vi "Get All Process Names.vi"(11 "?":T16 {"Main Config"."PR Module Configs"."Settings"."PID 2 Parameters"."output range"."output low" format="%.2f"; "Main Config"."PR Module Configs"."Settings"."PID 2 Parameters"."output range"."output high" min=0.0 max=100.0 format="%.2f"; "Main Config"."PR Module Configs"."Settings"."PID 2 Parameters"."PID gains"."derivative time (Td, min)" format="%.3f"; "Main Config"."PR Module Configs"."Settings"."PID 2 Parameters"."PID gains"."integral time (Ti, min)" format="%.3f"; "Main Config"."PR Module Configs"."Settings"."PID 2 Parameters"."PID gains"."proportional gain (Kc)" format="%.3f"; "Main Config"."Steps"."Control" items=["Pump %", "Setpoint"]; "Main Config"."TCU Module Configs"."Settings"."Huber Unistat 410 Settings"."Address" min=0 max=99 format="%02.0f"; "Main Config"."TCU Module Configs"."Settings"."Julabo FP-50 Settings"."Pump Power" min=0 max=8 step=1; "Main Config"."TCU Module Configs"."Settings"."Lauda Settings"."Pump Power" min=0 max=8 step=1; "Main Config"."Flow Module Configs"."Settings"."Bronkhorst M14 Settings"."Smoothing Steps" min=1 step=1; "Main Config"."Flow Module Configs"."Settings"."Bronkhorst M13 Settings"."Smoothing Steps" min=1 step=1; "Main Config"."Pump Module Configs"."Settings"."Ismatech 3 Channel Settings"."Channel Number" min=0 max=3; "Main Config"."Pump Module Configs"."Settings"."Ismatech 3 Channel Settings"."Pump Number" min=1; "Main Config"."Pump Module Configs"."Settings"."ASIA Pump C"."channel" min=0 max=1 step=1; "Main Config"."Pump Module Configs"."Settings"."Masterflex"."Pump Number" min=1.0 max=20.0 step=1.0; "Main Config"."Pump Module Configs"."Settings"."Ismatech"."Pump Number" min=1.0 max=20.0 step=1.0; "Main Config"."Feed Module Configs"."Settings"."Bronkhorst M14 Settings"."Smoothing Steps" min=1 step=1; "Main Config"."Feed Module Configs"."Settings"."Ismatech 3 Channel Settings"."Channel Number" min=0 max=3; "Main Config"."Feed Module Configs"."Settings"."Ismatech 3 Channel Settings"."Pump Number" min=1; "Main Config"."Feed Module Configs"."Settings"."PID range"."PID Low" min=0.0 max=100.0 format="%.2f"; "Main Config"."Feed Module Configs"."Settings"."PID range"."PID High" format="%.2f"; "Main Config"."Feed Module Configs"."Settings"."PID 2 Parameters"."PID gains"."derivative time (Td, min)" format="%.3f"; "Main Config"."Feed Module Configs"."Settings"."PID 2 Parameters"."PID gains"."integral time (Ti, min)" format="%.3f"; "Main Config"."Feed Module Configs"."Settings"."PID 2 Parameters"."PID gains"."proportional gain (Kc)" format="%.3f"; "Main Config"."Feed Module Configs"."Settings"."Bronkhorst M13 Flow Meter"."Smoothing Steps" min=1 step=1; "Main Config"."Feed Module Configs"."Settings"."ASIA Pump C"."channel" min=0 max=1 step=1; "Main Config"."Feed Module Configs"."Settings"."Ismatech"."Pump Number" min=1.0 max=20.0 step=1.0; "Main Config"."Feed Module Configs"."Settings"."Masterflex"."Pump Number" min=1.0 max=20.0 step=1.0}) -> (2 "Module Strings":T3, 3 "Module Tags Array Cluster":T6)   [LabVIEW 2018, in "OPC UA.lvlib"]
uses:
  OPC/OPC UA.lvlib
  Drag and Drop/State Cluster.ctl
  Message Queue/Message Cluster.ctl
  Drag and Drop/Thumbnail Cluster.ctl
  Drag and Drop/Object Cluster.ctl
  <vilib>/Utility/miscctls.llb/LVRectTypeDef.ctl
  Drag and Drop/Object Type Enum.ctl
  <vilib>/Utility/miscctls.llb/LVPositionTypeDef.ctl
  Config Module/Controls/Main Config Cluster.ctl
  OPC/OPC Module Config.ctl
  Scale Module Folder/Measure Instrument/State Enum.ctl
  <vilib>/Utility/miscctls.llb/LVPoint32TypeDef.ctl
  OPC/OPC Settings.ctl
  OPC/Variable Data Cluster.ctl
  <vilib>/OPCUA/controls/NodeId.ctl
  <vilib>/OPCUA/controls/OPC UA StatusCode.ctl
  <vilib>/OPCUA/controls/Subscription ID.ctl
  <vilib>/OPCUA/controls/OPC UA Client Refnum.ctl
  <vilib>/OPCUA/controls/Subscription Data Change.ctl
  <vilib>/OPCUA/controls/Data Type.ctl
  OPC/OPC Tag Data.ctl
  Feed Module/Controls/Feed Module Config Cluster.ctl
  Feed Module/Controls/Feed Module Settings Cluster.ctl
  Ismatec ISM 831C/Controls/Ismatech ISM831C Settings Cluster.ctl
  Masterflex 7550-30/Controls/Settings Cluster.ctl
  Mettler Toledo/Controls/Settings Cluster.ctl
  Bronkhorst M13 Flow Meter/Settings Cluster.ctl
  Measure Instrument/PID 2 Parameters Cluster.ctl
  Measure Instrument/PID Input Enum.ctl
  Measure Instrument/PID 2 Output Enum.ctl
  Tacmina QI/Tacmina QI DAQ Setting.ctl
  KNF Pump/Settings Cluster plus SIMDOS.ctl
  ASIA Pump/Pump Settings.ctl
  VICI M50 Party Mode/Settings Cluster.ctl
  FLOM Pump/Settings Cluster.ctl
  SSI PR Class/SSI PR or LD Settings Cluster.ctl
  Masterflex 75211/Masterflex 75211 DAQ Setting.ctl
  SSI PR Class/SSI P40 Settings Cluster.ctl
  Ismatec 78001/Ismatec 4083.ctl
  Bronkhorst M14 Flow Meter/Settings Cluster.ctl
  Tag VIs/Numeric Alarm Settings Cluster.ctl
  TT Module/Controls/TT Module Config Cluster.ctl
  Acquisition/Hardware Configuration.ctl
  Acquisition/Task Cluster.ctl
  PT Module/Controls/PT Module Config Cluster.ctl
  Scale Module Folder/Feed Module/Controls/Scale Module Config Cluster.ctl
  Scale Module Folder/Feed Module/Controls/Scale Module Settings Cluster.ctl
  Pump Module Folder/Pump Module Config Cluster.ctl
  Pump Module Folder/Pump Module Settings Cluster.ctl
  LabJack Module/Controls/U3 Module Config Cluster.ctl
  Decoration Module/Decoration Module Config Cluster.ctl
  Flow Module Folder/Feed Module/Controls/Flow Module Config Cluster.ctl
  Flow Module Folder/Feed Module/Controls/Flow Module Settings Cluster.ctl
  TCU Module/TCU Module Folder/TCU Module Config Cluster.ctl
  TCU Module/TCU Module Folder/TCU Module Settings Cluster.ctl
  TCU Module/TCU Module Folder/Measure Instrument/Output Devices.ctl
  Huber TCU/Huber Settings.ctl
  Lauda Integral XT-150 TCU/Lauda Settings.ctl
  Julabo Type 1 TCU/Julabo Type 1 TCU Folder/Julabo FP-50 Settings.ctl
  Huber Unistat 410 TCU/Huber Unistat 410 RS485 Settings.ctl
  D-O Module Folder/Not Sure Where this is Used.ctl
  Sequencing/Squence Control.ctl
  D-O Module Folder/D-O Module Config Cluster.ctl
  D-O Module Folder/Valve Clusters.ctl
  D-O Module Folder/D-O Module Settings Cluster.ctl
  D-O Module Folder/D-O Device Settings Cluster.ctl
  VICI Electronic Actuator/VICI Electronic Actuator Settings.ctl
  Pressure Regulator Control Module/Pressure Regulator/Controls/4-20mA Module Config Cluster.ctl
  Pressure Regulator Control Module/Pressure Regulator/Controls/4-20mA Module Settings Cluster.ctl
  Pressure Transmitter/Pressure Transmitter Device Settings.ctl
  Pressure Reg Module/Pressure Regulator Device Settings.ctl
  Sonicator Module Folder/Feed Module/Controls/Sonicator Module Config Cluster.ctl
  Sonicator Module Folder/Feed Module/Controls/Sonicator Module Settings Cluster.ctl
  Sonic Systems P100/Sonic Systems P100 Settings.ctl
  Agitator Module Folder/Feed Module/Controls/Agitator Module Config Cluster.ctl
  Agitator Module Folder/Feed Module/Controls/Agitator Module Settings Cluster.ctl
  IKA EUROSTAR/IKA EUROSTAR Settings.ctl
  Centrifuge Module Folder/Centrifuge Module Config Cluster.ctl
  Centrifuge Module Folder/Centrifuge Module Settings Cluster.ctl
  EPOS4/Controls/Device Selection.ctl
  EPOS4/Controls/EPOS Communication Settings.ctl
  Feed Module/Controls/Feed Module Tag Names Cluster.ctl
  Pump Module Folder/Pump Module Tag Names Cluster.ctl
  Bronkhorst M14 Flow Meter/Tag Cluster.ctl
  TCU Module/TCU Module Folder/TCU Module Tag Names Cluster.ctl
  Pressure Regulator Control Module/Pressure Regulator/Controls/4-20mA Module Tag Names Cluster.ctl
  OPC/OPC Module Tag Names.ctl
  OPC/Module Tags Array Cluster.ctl
  TT Module/Controls/TT Module Tag Names.ctl
  PT Module/Controls/PT Module Tag Names.ctl
  D-O Module Folder/D-O Module Tag Names Cluster.ctl
  Sonicator Module Folder/Feed Module/Controls/Sonicator Module Tag Names.ctl
  Agitator Class/Agitator Module Tag Names.ctl
  Centrifuge Module Folder/Centrifuge Module Tag Names Cluster.ctl
  TT Module/TT Module.lvlib
  PT Module/PT Module.lvlib
  D-O Module Folder/D-O Module.lvlib
  Agitator Module Folder/Agitator Module.lvlib
  Sonicator Module Folder/Sonicator Module.lvlib
  Pressure Regulator Control Module/Pressure Regulator/4-20mA Module.lvlib
  TCU Module/TCU Module Folder/TCU Module.lvlib
  Flow Module Folder/Flow Module.lvlib
  Pump Module Folder/Pump Module.lvlib
  Feed Module/Feed Module.lvlib
  <resource>/objmgr/daqmx.rc
  Centrifuge Module Folder/Centrifuge Module.lvlib
  Message Queue/Message Queue.lvlib
  Masterflex 7550-30/Masterflex 7550-30.lvlib
  Ismatec ISM 831C/Ismatec ISM 831C.lvlib
  Tacmina QI/Tacmina QI.lvlib
  KNF Pump/KNF SIMDOS.lvlib
  VICI M50 Party Mode/VICI M6 M50 Party Mode.lvlib
  FLOM Pump/FLOM Pump.lvlib
  ASIA Pump.lvlib
  Mettler Toledo/Mettler Toledo.lvlib
  Bronkhorst M13 Flow Meter/Bronkhorst M13 Flow Meter.lvlib
  SSI PR Class/SSI PR or LD Pump.lvlib
  DAQ/DAQ.lvlib
  Scale Module Folder/Scale Module.lvlib
  LabJack Module/U3 Module.lvlib
  Huber TCU/Huber Ministat 230 TCU.lvlib
  Lauda Integral XT-150 TCU/Lauda TCU.lvlib
  Julabo Type 1 TCU/Julabo Type 1 TCU Folder/Julabo Type FP-50 TCU.lvlib
  Sequencing/Sequencing Library.lvlib
  Pressure Transmitter/Pressure Transmitter Library.lvlib
  Pressure Reg Module/Pressure Regulator Library.lvlib
  Scale Module Folder/Measure Instrument/Scale Module Engine.lvlib
  Config Module/Config Module.lvlib
  Drag and Drop/Drag and Drop.lvlib
  D-O Module Folder/DIO Valve/VICI Electronic Actuator.lvlib
  Masterflex 75211/Masterflex 75211.lvlib
  SSI PR Class/SSI P40 Pump.lvlib
  Huber Unistat 410 TCU/Huber Unistat 410 TCU.lvlib
  Ismatec 78001/Ismatec 4308.lvlib
  Bronkhorst M14 Flow Meter/Bronkhorst M14 Flow Meter.lvlib
  Sonic Systems P100/Sonic Systems P100.lvlib
  EPOS4/EPOS4.lvlib
  IKA EUROSTAR/IKA EUROSTAR.lvlib
panel:
  out "CM Module Tags Array":T1[](array[typedef])
  out "Scale Tags Array":T2(array[cluster])
  out "AM Module Tags Array":T4[](array[typedef])
  out "Sonicator Module Tags Array":T5[](array[typedef])
  out "OPC Array":T15[](array[typedef])
  out "PR Array":T14[](array[typedef])
  out "TCU Array":T12[](array[typedef])
  out "Flow Array":T11[](array[typedef])
  out "Pump Array":T10[](array[typedef])
  out "DAQ Array":string[](array[string])
  out "Feed Module Array":T7[](array[typedef])
  out "output array":string[](array[string])
  out "appended array":string[][](array[string])
  # "Agitator Settings"
  # "Sonicator Settings"
  # "Instrument Settings"
  # "Instrument Settings"
  # "Output Instruments"
  # "Flow Meter Settings"
  # "Output Instruments"
  # "Scale Settings"
  # "Output Instruments"
  # "Input Instruments"
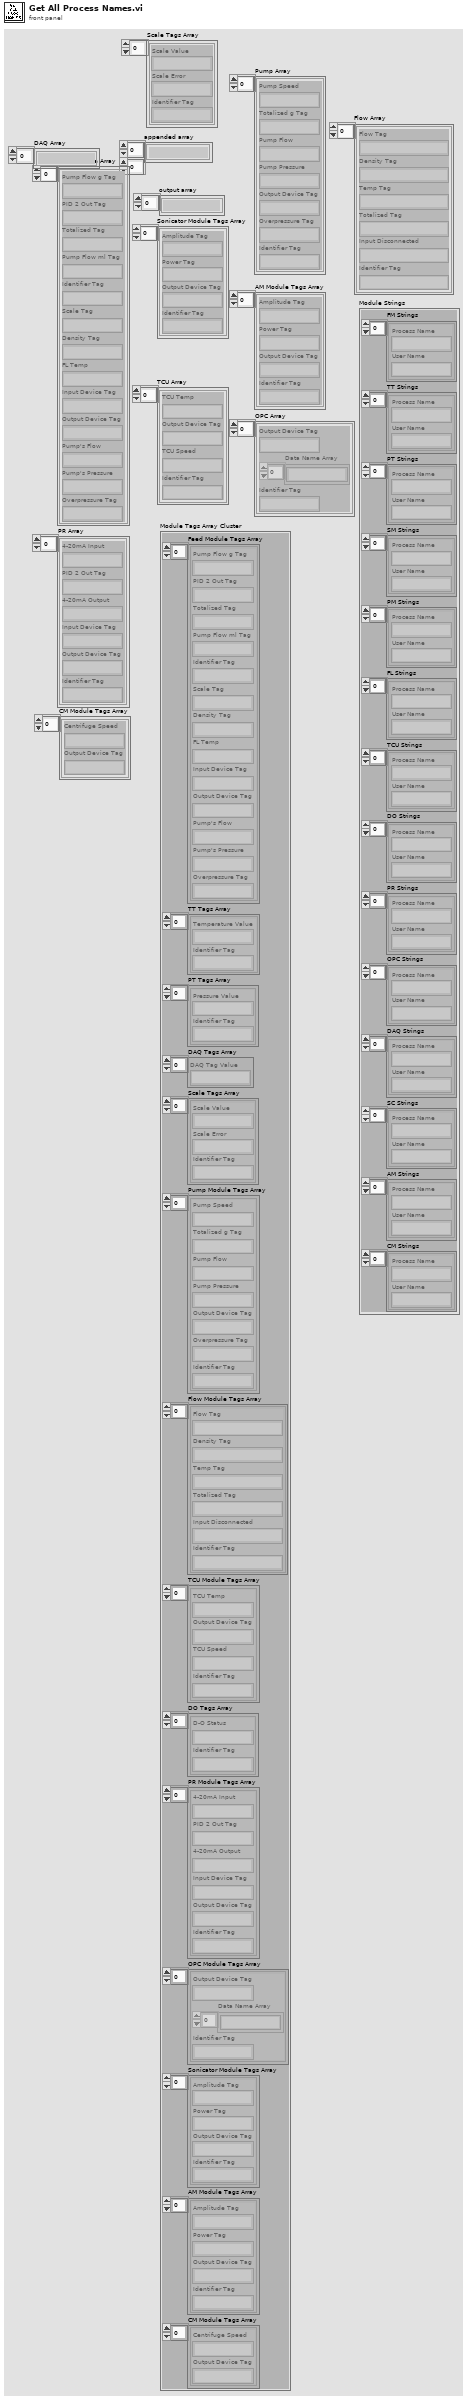
[diagram p1: front panel]
types:
  T1 = typedef "Centrifuge Module.lvlib/Centrifuge Module Tag Names Cluster.ctl" = cluster{"Centrifuge Speed":string, "Output Device Tag":string}
  T2 = cluster{"Scale Value":string, "Scale Error":string, "Identifier Tag":string}[]
  T3 = cluster{"FM Strings":cluster{"Process Name":string, "User Name":string}[], "TT Strings":cluster{"Process Name":string, "User Name":string}[], "PT Strings":cluster{"Process Name":string, "User Name":string}[], "SM Strings":cluster{"Process Name":string, "User Name":string}[], "PM Strings":cluster{"Process Name":string, "User Name":string}[], "FL Strings":cluster{"Process Name":string, "User Name":string}[], "TCU Strings":cluster{"Process Name":string, "User Name":string}[], "DO Strings":cluster{"Process Name":string, "User Name":string}[], "PR Strings":cluster{"Process Name":string, "User Name":string}[], "OPC Strings":cluster{"Process Name":string, "User Name":string}[], "DAQ Strings":cluster{"Process Name":string, "User Name":string}[], "SC Strings":cluster{"Process Name":string, "User Name":string}[], "AM Strings":cluster{"Process Name":string, "User Name":string}[], "CM Strings":cluster{"Process Name":string, "User Name":string}[]}
  T4 = typedef "Agitator Module.lvlib/Agitator Module Tag Names.ctl" = cluster{"Amplitude Tag":string, "Power Tag":string, "Output Device Tag":string, "Identifier Tag":string}
  T5 = typedef "Sonicator Module.lvlib/Sonicator Module Tag Names.ctl" = cluster{"Amplitude Tag":string, "Power Tag":string, "Output Device Tag":string, "Identifier Tag":string}
  T6 = typedef "Module Tags Array Cluster.ctl" = cluster{"Feed Module Tags Array":T7[], "TT Tags Array":T8[], "PT Tags Array":T9[], "DAQ Tags Array":string[], "Scale Tags Array":cluster{"Scale Value":string, "Scale Error":string, "Identifier Tag":string}[], "Pump Module Tags Array":T10[], "Flow Module Tags Array":T11[], "TCU Module Tags Array":T12[], "DO Tags Array":T13[], "PR Module Tags Array":T14[], "OPC Module Tags Array":T15[], "Sonicator Module Tags Array":T5[], "AM Module Tags Array":T4[], "CM Module Tags Array":T1[]}
  T7 = typedef "Feed Module.lvlib/Feed Module Tag Names Cluster.ctl" = cluster{"Pump Flow g Tag":string, "PID 2 Out Tag":string, "Totalized Tag":string, "Pump Flow ml Tag":string, "Identifier Tag":string, "Scale Tag":string, "Density Tag":string, "FL Temp":string, "Input Device Tag":string, "Output Device Tag":string, "Pump's Flow":string, "Pump's Pressure":string, "Overpressure Tag":string}
  T8 = typedef "TT Module.lvlib/TT Module Tag Names.ctl" = cluster{"Temperature Value":string, "Identifier Tag":string}
  T9 = typedef "PT Module.lvlib/PT Module Tag Names.ctl" = cluster{"Pressure Value":string, "Identifier Tag":string}
  T10 = typedef "Pump Module.lvlib/Pump Module Tag Names Cluster.ctl" = cluster{"Pump Speed":string, "Totalized g Tag":string, "Pump Flow":string, "Pump Pressure":string, "Output Device Tag":string, "Overpressure Tag":string, "Identifier Tag":string}
  T11 = typedef "Flow Module.lvlib/Tag Cluster.ctl" = cluster{"Flow Tag":string, "Density Tag":string, "Temp Tag":string, "Totalized Tag":string, "Input Disconnected":string, "Identifier Tag":string}
  T12 = typedef "TCU Module.lvlib/TCU Module Tag Names Cluster.ctl" = cluster{"TCU Temp":string, "Output Device Tag":string, "TCU Speed":string, "Identifier Tag":string}
  T13 = typedef "D-O Module.lvlib/D-O Module Tag Names Cluster.ctl" = cluster{"D-O Status":string, "Identifier Tag":string}
  T14 = typedef "4-20mA Module.lvlib/4-20mA Module Tag Names Cluster.ctl" = cluster{"4-20mA Input":string, "PID 2 Out Tag":string, "4-20mA Output":string, "Input Device Tag":string, "Output Device Tag":string, "Identifier Tag":string}
  T15 = typedef "OPC Module Tag Names.ctl" = cluster{"Output Device Tag":string, "Data Name Array":string[], "Identifier Tag":string}
  T16 = typedef "Drag and Drop.lvlib/State Cluster.ctl" = cluster{"VI refs":refnum<vi>[], "Queues":refnum<queue>[], "[Thumbnails]":T17[], "Drag Object Idx":i32, "[Objects]":T18[], "Active Object":i32, "Drop Offset":T21, "Process Name":string, "Main Config":T22, "Campaign Filepath":path, "Config Changed?":bool}
  T17 = typedef "Thumbnail Cluster.ctl" = cluster{"Path":path, "Rectangle":cluster{"left":i16, "top":i16, "right":i16, "bottom":i16}}
  T18 = typedef "Object Cluster.ctl" = cluster{"BMP Path":path, "Anchor Position":cluster{"X":i32, "Y":i32}, "Hot Spot":T19, "Type":T20, "Parameters":variant}
  T19 = typedef "LVRectTypeDef.ctl" = cluster{"Left":i16, "Top":i16, "Right":i16, "Bottom":i16}
  T20 = typedef "Object Type Enum.ctl" = enum16{"Icon", "Line", "Text", "Feed Module"}
  T21 = typedef "LVPositionTypeDef.ctl" = cluster{"Left":i32, "Top":i32}
  T22 = typedef "Config Module.lvlib/Main Config Cluster.ctl" = cluster{"Notebook":string, "OPC Module Configs":T23[], "Feed Module Configs":T33[], "Log File Path":path, "TT Module Configs":T53[], "DAQ Config":T54, "PT Module Configs":T56[], "Scale Module Configs":T57[], "Pump Module Configs":T59[], "U3 Module Configs":T61[], "Decoration Module Configs":T62[], "Flow Module Configs":T63[], "TCU Module Configs":T65[], "Steps":T72, "Abort":bool, "DO Module Configs":T74[], "PR Module Configs":T79[], "SC Module Configs":T83[], "AM Module Configs":T86[], "CM Module Configs":T89[], "Cycle Period":dbl}
  T23 = typedef "OPC UA.lvlib/OPC Module Config.ctl" = cluster{"State":T24, "GUID":string, "Process Name":string, "User name":string, "Drop Coords":T25, "Configuration":T26, "First Iteration":bool, "Data":cluster{"Object Name":string, "Variable Array":T27[]}[], "Load Count":i32, "Log Started":bool, "subscription ID out":T30, "OPC UA client refnum out":T31, "Event Registration Refnum":refnum<event-registration>, "Start Time":timestamp, "Current Time":timestamp, "Tag Data":T32[]}
  T24 = typedef "Scale Module.lvlib/Scale Module Engine.lvlib/State Enum.ctl" = enum16{"Measuring", "Idle"}
  T25 = typedef "LVPoint32TypeDef.ctl" = cluster{"Horizontal":i32, "Vertical":i32}
  T26 = typedef "OPC UA.lvlib/OPC Settings.ctl" = cluster{"Cycle Period":dbl, "server endpoint URL":string, "security policy":cluster{"message mode":enum16{"None", "Sign", "Sign and Encrypt"}, "security":enum16{"Basic256", "Basic128Rsa15"}}, "Trust Any Server":bool}
  T27 = typedef "OPC UA.lvlib/Variable Data Cluster.ctl" = cluster{"node ID":T28, "browse name":string, "status":T29, "timestamp":timestamp, "value ":variant}
  T28 = typedef "NodeId.ctl" = string
  T29 = typedef "OPC UA StatusCode.ctl" = u32
  T30 = typedef "Subscription ID.ctl" = u32
  T31 = typedef "OPC UA Client Refnum.ctl" = refnum<k21>
  T32 = typedef "OPC UA.lvlib/OPC Tag Data.ctl" = cluster{"Include this Device":bool, "Device Name":string, "OPC Tag Data":cluster{"Tag":string, "Value":variant, "Time Stamp":timestamp}[]}
  T33 = typedef "Feed Module.lvlib/Feed Module Config Cluster.ctl" = cluster{"GUID":string, "Drop Coords":T25, "Process Name":string, "User name":string, "Queue Name":string, "Settings":T34, "Settings Load Count":i32, "OP Load Count":i32}
  T34 = typedef "Feed Module.lvlib/Feed Module Settings Cluster.ctl" = cluster{"Cycle Period":dbl, "Ismatech":T35, "Masterflex":T36, "Mettler":T37, "Bronkhorst M13 Flow Meter":T38, "PID 2 Parameters":T39, "Manual Entry":dbl, "Auto?":bool, "PID range":cluster{"PID High":dbl, "PID Low":dbl, "High Warning":dbl}, "Tacmina Settings":T42, "KNF SIMDOS Settings":T43, "ASIA Pump C":T44, "VICI Settings":T45, "FLOM Settings":T46, "SSI PR/LD Settings":T47, "Masterflex 75211 Settings":T48, "SSI P40 Settings":T49, "Ismatech 3 Channel Settings":T50, "Bronkhorst M14 Settings":T51, "Reset Totalizer":bool, "Input Num Alarm Settings":T52[], "Control Type":enum32{"g/min", "ml/min"}, "Front End Display Options":cluster{"Temperature":bool, "Scale Grams":bool, "Density":bool, "Flow (g/min)":bool, "Flow (ml/min)":bool, "PSIG":bool, "Total Grams":bool, "Updated":bool}}
  T35 = typedef "Ismatec ISM 831C.lvlib/Ismatech ISM831C Settings Cluster.ctl" = cluster{"VISA resource name":refnum<visa-resource-name>, "Simulated?":bool, "Pump Number":dbl, "Reverse?":bool}
  T36 = typedef "Masterflex 7550-30.lvlib/Settings Cluster.ctl" = cluster{"VISA resource name":refnum<visa-resource-name>, "Simulated?":bool, "Pump Number":dbl, "Reverse?":bool}
  T37 = typedef "Mettler Toledo.lvlib/Settings Cluster.ctl" = cluster{"VISA resource name":refnum<visa-resource-name>, "Simulated?":bool}
  T38 = typedef "Bronkhorst M13 Flow Meter.lvlib/Settings Cluster.ctl" = cluster{"VISA resource name":refnum<visa-resource-name>, "Simulated?":bool, "Smoothing Steps":i32}
  T39 = typedef "PID 2 Parameters Cluster.ctl" = cluster{"Input Device":T40, "Output Device":T41, "Setpoint":dbl, "PID gains":cluster{"proportional gain (Kc)":dbl, "integral time (Ti, min)":dbl, "derivative time (Td, min)":dbl}}
  T40 = typedef "PID Input Enum.ctl" = enum16{"Default", "Bronkhorst M13", "Bronkhorst M14", "Scale Rate of Change"}
  T41 = typedef "PID 2 Output Enum.ctl" = enum16{"Default", "Ismatec ISM 4308", "Ismatec ISM 831C", "Masterflex 7550-30", "VICI M6", "VICI M50", "Tacmina QI", "KNF SIMDOS", "ASIA Type C", "FLOM UI-22-11", "SSI PR/LD", "SSI P40", "Masterflex 75211-70"}
  T42 = typedef "Tacmina QI.lvlib/Tacmina QI DAQ Setting.ctl" = cluster{"Analog DAQ Task":refnum<k21>, "Digital DAQ Task":refnum<k21>}
  T43 = typedef "KNF SIMDOS.lvlib/Settings Cluster plus SIMDOS.ctl" = cluster{"VISA resource name":refnum<visa-resource-name>, "Simulated?":bool}
  T44 = typedef "ASIA Pump.lvlib/Pump Settings.ctl" = cluster{"ASIA Pump #":i32, "channel":i32, "Simulated":bool}
  T45 = typedef "VICI M6 M50 Party Mode.lvlib/Settings Cluster.ctl" = cluster{"VISA resource name":refnum<visa-resource-name>, "Pump ID":string, "Pump Head Vol":dbl, "Reverse?":bool, "Simulated?":bool}
  T46 = typedef "FLOM Pump.lvlib/Settings Cluster.ctl" = cluster{"VISA resource name":refnum<visa-resource-name>, "Simulated?":bool, "Pump Number":dbl}
  T47 = typedef "SSI PR or LD Pump.lvlib/SSI PR or LD Settings Cluster.ctl" = cluster{"VISA resource name":refnum<visa-resource-name>, "Simulated?":bool}
  T48 = typedef "Masterflex 75211.lvlib/Masterflex 75211 DAQ Setting.ctl" = cluster{"Analog DAQ Task":refnum<k21>, "Digital DAQ Task":refnum<k21>}
  T49 = typedef "SSI P40 Pump.lvlib/SSI P40 Settings Cluster.ctl" = cluster{"VISA resource name":refnum<visa-resource-name>, "Simulated?":bool}
  T50 = typedef "Ismatec 4308.lvlib/Ismatec 4083.ctl" = cluster{"VISA resource name":refnum<visa-resource-name>, "Pump Number":i16, "Channel Number":i16, "Simulated?":bool, "Reverse?":bool}
  T51 = typedef "Bronkhorst M14 Flow Meter.lvlib/Settings Cluster.ctl" = cluster{"VISA resource name":refnum<visa-resource-name>, "Simulated?":bool, "Smoothing Steps":i32}
  T52 = typedef "Numeric Alarm Settings Cluster.ctl" = cluster{"enable? (F)":bool, "name":string, "alarm type":enum16{"HI_HI", "HI", "LO", "LO_LO"}, "level/change":dbl, "deadband/time":dbl, "alarm delay":dbl, "priority":u32, "ack type":enum16{"Auto", "User", "None", "Each Occurrence"}, "area":string, "description":string, "log? (T)":bool}
  T53 = typedef "TT Module.lvlib/TT Module Config Cluster.ctl" = cluster{"GUID":string, "Drop Coords":T25, "Input Channel Tag Name ":string, "Process Name":string, "User name":string, "Queue Name":string, "Input Channel Numeric Alarm Settings":T52[]}
  T54 = typedef "DAQ.lvlib/Hardware Configuration.ctl" = cluster{"Tasks Array":T55[]}
  T55 = typedef "Task Cluster.ctl" = cluster{"DAQmx Task":refnum<k21>, "Read-Write Radio":enum32{"Read", "Write"}}
  T56 = typedef "PT Module.lvlib/PT Module Config Cluster.ctl" = cluster{"GUID":string, "Drop Coords":T25, "Input Channel Tag Name ":string, "Process Name":string, "User name":string, "Queue Name":string, "Input Channel Numeric Alarm Settings":T52[]}
  T57 = typedef "Scale Module.lvlib/Scale Module Config Cluster.ctl" = cluster{"GUID":string, "Drop Coords":T25, "Process Name":string, "User name":string, "Queue Name":string, "Settings":T58, "Load Count":i32}
  T58 = typedef "Scale Module.lvlib/Scale Module Settings Cluster.ctl" = cluster{"Cycle Period":dbl, "Mettler":T37, "Scale Type":string}
  T59 = typedef "Pump Module.lvlib/Pump Module Config Cluster.ctl" = cluster{"GUID":string, "Drop Coords":T25, "Process Name":string, "User name":string, "Queue Name":string, "Settings":T60, "Load Count":i32}
  T60 = typedef "Pump Module.lvlib/Pump Module Settings Cluster.ctl" = cluster{"Cycle Period":dbl, "Manual Entry":dbl, "Output Device":T41, "Ismatech":T35, "Ismatech 3 Channel Settings":T50, "Masterflex":T36, "VICI Settings":T45, "Tacmina Settings":T42, "KNF SIMDOS Settings":T43, "ASIA Pump C":T44, "FLOM Settings":T46, "SSI PR/LD Settings":T47, "SSI P40 Settings":T47, "Masterflex 75211 Settings":T48, "Pump Calibration File":path, "Calibration Slope":dbl, "Calibration Y Intercept":dbl, "Pump Cal Enum":u16, "Reset Totalizer":bool}
  T61 = typedef "U3 Module.lvlib/U3 Module Config Cluster.ctl" = cluster{"GUID":string, "Drop Coords":T25, "AI Channel Number":enum16{"Default", "AI0", "AI1", "AI2", "AI3", "AI4", "AI5", "AI6", "AI7"}, "Process Name":string, "User name":string, "Queue Name":string, "Input Channel Numeric Alarm Settings":T52[]}
  T62 = typedef "Decoration Module Config Cluster.ctl" = cluster{"GUID":string, "Drop Coords":T25, "Decoration Filepath":path}
  T63 = typedef "Flow Module.lvlib/Flow Module Config Cluster.ctl" = cluster{"GUID":string, "Drop Coords":T25, "Process Name":string, "User name":string, "Queue Name":string, "Settings":T64, "Load Count":i32}
  T64 = typedef "Flow Module.lvlib/Flow Module Settings Cluster.ctl" = cluster{"Cycle Period":dbl, "Flow Meter Type":string, "Bronkhorst M13 Settings":T38, "Bronkhorst M14 Settings":T51, "Reset Totalizer":bool}
  T65 = typedef "TCU Module.lvlib/TCU Module Config Cluster.ctl" = cluster{"GUID":string, "Drop Coords":T25, "Process Name":string, "User name":string, "Queue Name":string, "Settings":T66, "Load Count":i32, "Power Level Changed":bool}
  T66 = typedef "TCU Module.lvlib/TCU Module Settings Cluster.ctl" = cluster{"Cycle Period":dbl, "Setpoint Entry":dbl, "Output Device":T67, "Huber Ministat 230 Settings":T68, "Lauda Settings":T69, "Julabo FP-50 Settings":T70, "Internal Control?":bool, "Huber Unistat 410 Settings":T71}
  T67 = typedef "Output Devices.ctl" = enum16{"Default", "Huber Ministat 230", "Huber Unistat 410", "Lauda XT-150", "Julabo FP-50"}
  T68 = typedef "Huber Ministat 230 TCU.lvlib/Huber Settings.ctl" = cluster{"VISA resource name":refnum<visa-resource-name>, "Simulated?":bool}
  T69 = typedef "Lauda TCU.lvlib/Lauda Settings.ctl" = cluster{"VISA resource name":refnum<visa-resource-name>, "Simulated?":bool, "Pump Power":i32}
  T70 = typedef "Julabo Type FP-50 TCU.lvlib/Julabo FP-50 Settings.ctl" = cluster{"VISA resource name":refnum<visa-resource-name>, "Simulated?":bool, "Pump Power":i32}
  T71 = typedef "Huber Unistat 410 TCU.lvlib/Huber Unistat 410 RS485 Settings.ctl" = cluster{"VISA resource name":refnum<visa-resource-name>, "Address":i8, "Simulated?":bool}
  T72 = typedef "Not Sure Where this is Used.ctl" = T73[]
  T73 = typedef "Sequencing Library.lvlib/Squence Control.ctl" = cluster{"Module":string, "Control":u16, "Value":dbl, "Wait (sec)":dbl}
  T74 = typedef "D-O Module.lvlib/D-O Module Config Cluster.ctl" = cluster{"GUID":string, "Drop Coords":T25, "Process Name":string, "User name":string, "Queue Name":string, "Settings":T75, "Load Count":i32}
  T75 = typedef "D-O Module.lvlib/Valve Clusters.ctl" = cluster{"Valve Settings":T76, "Valve Type":enum16{"Default", "Digital Output Valve", "VICI Electronic Actuator"}, "Time On (Sec)":dbl, "Time Off (Sec)":dbl, "Run?":bool}
  T76 = typedef "D-O Module.lvlib/D-O Module Settings Cluster.ctl" = cluster{"D-O Settings":T77, "VICI Electronic Actuator":T78}
  T77 = typedef "D-O Module.lvlib/D-O Device Settings Cluster.ctl" = cluster{"DAQmx Task Name":refnum<k21>, "Output Channel":u16, "Output Channel Names":string[]}
  T78 = typedef "VICI Electronic Actuator.lvlib/VICI Electronic Actuator Settings.ctl" = cluster{"VISA resource name":refnum<visa-resource-name>, "Mode":enum16{"Two Positions With Stops", "Two Positions Without Stops", "Mutiposition"}, "Simulated":bool}
  T79 = typedef "4-20mA Module.lvlib/4-20mA Module Config Cluster.ctl" = cluster{"GUID":string, "Drop Coords":T25, "Process Name":string, "User name":string, "Queue Name":string, "Settings":T80, "Settings Load Count":i32}
  T80 = typedef "4-20mA Module.lvlib/4-20mA Module Settings Cluster.ctl" = cluster{"Cycle Period":dbl, "PID 2 Parameters":cluster{"Input Device":enum16{"Default", "4-20mA"}, "Output Device":enum16{"Default", "Equilibar Pressure Reg", "Flow Regulator"}, "Setpoint":dbl, "PID gains":cluster{"proportional gain (Kc)":dbl, "integral time (Ti, min)":dbl, "derivative time (Td, min)":dbl}, "output range":cluster{"output low":dbl, "output high":dbl}}, "Manual Entry":dbl, "Auto?":bool, "4-20mA Input Settings":T81, "4-20mA Out Settings":T82, "Input Channel Tag Name ":string}
  T81 = typedef "Pressure Transmitter Library.lvlib/Pressure Transmitter Device Settings.ctl" = cluster{"Input Channel ":u16}
  T82 = typedef "Pressure Regulator Library.lvlib/Pressure Regulator Device Settings.ctl" = cluster{"Output DAQ Task":refnum<k21>}
  T83 = typedef "Sonicator Module.lvlib/Sonicator Module Config Cluster.ctl" = cluster{"GUID":string, "Drop Coords":T25, "Process Name":string, "User name":string, "Queue Name":string, "Settings":T84, "Load Count":i32}
  T84 = typedef "Sonicator Module.lvlib/Sonicator Module Settings Cluster.ctl" = cluster{"Cycle Period":dbl, "Sonicator Type":string, "SS P100 Settings":T85, "Setpoint (µm)":dbl, "Cutoff (W)":dbl}
  T85 = typedef "Sonic Systems P100.lvlib/Sonic Systems P100 Settings.ctl" = cluster{"VISA resource name":refnum<visa-resource-name>, "Simulated?":bool}
  T86 = typedef "Agitator Module.lvlib/Agitator Module Config Cluster.ctl" = cluster{"GUID":string, "Drop Coords":T25, "Process Name":string, "User name":string, "Queue Name":string, "Settings":T87, "Load Count":i32}
  T87 = typedef "Agitator Module.lvlib/Agitator Module Settings Cluster.ctl" = cluster{"Cycle Period":dbl, "Agitator Type":string, "Setpoint (µm)":dbl, "IKA EUROSTAR Settings":T88}
  T88 = typedef "IKA EUROSTAR.lvlib/IKA EUROSTAR Settings.ctl" = cluster{"VISA resource name":refnum<visa-resource-name>, "Simulated?":bool}
  T89 = typedef "Centrifuge Module.lvlib/Centrifuge Module Config Cluster.ctl" = cluster{"GUID":string, "Drop Coords":T25, "Process Name":string, "User name":string, "Queue Name":string, "Settings":T90, "Load Count":i32}
  T90 = typedef "Centrifuge Module.lvlib/Centrifuge Module Settings Cluster.ctl" = cluster{"Cycle Period":dbl, "Manual Entry":dbl, "Output Device":T91, "EPOS4 Settings":T92}
  T91 = typedef "Device Selection.ctl" = enum16{"Default", "EPOS4"}
  T92 = typedef "EPOS4.lvlib/EPOS Communication Settings.ctl" = cluster{"VISA resource name":refnum<visa-resource-name>, "axis":cluster{"keyHandle":u32, "nodeId":u16}, "Simulated?":bool}
  T93 = cluster{"Process Name":string, "User Name":string}
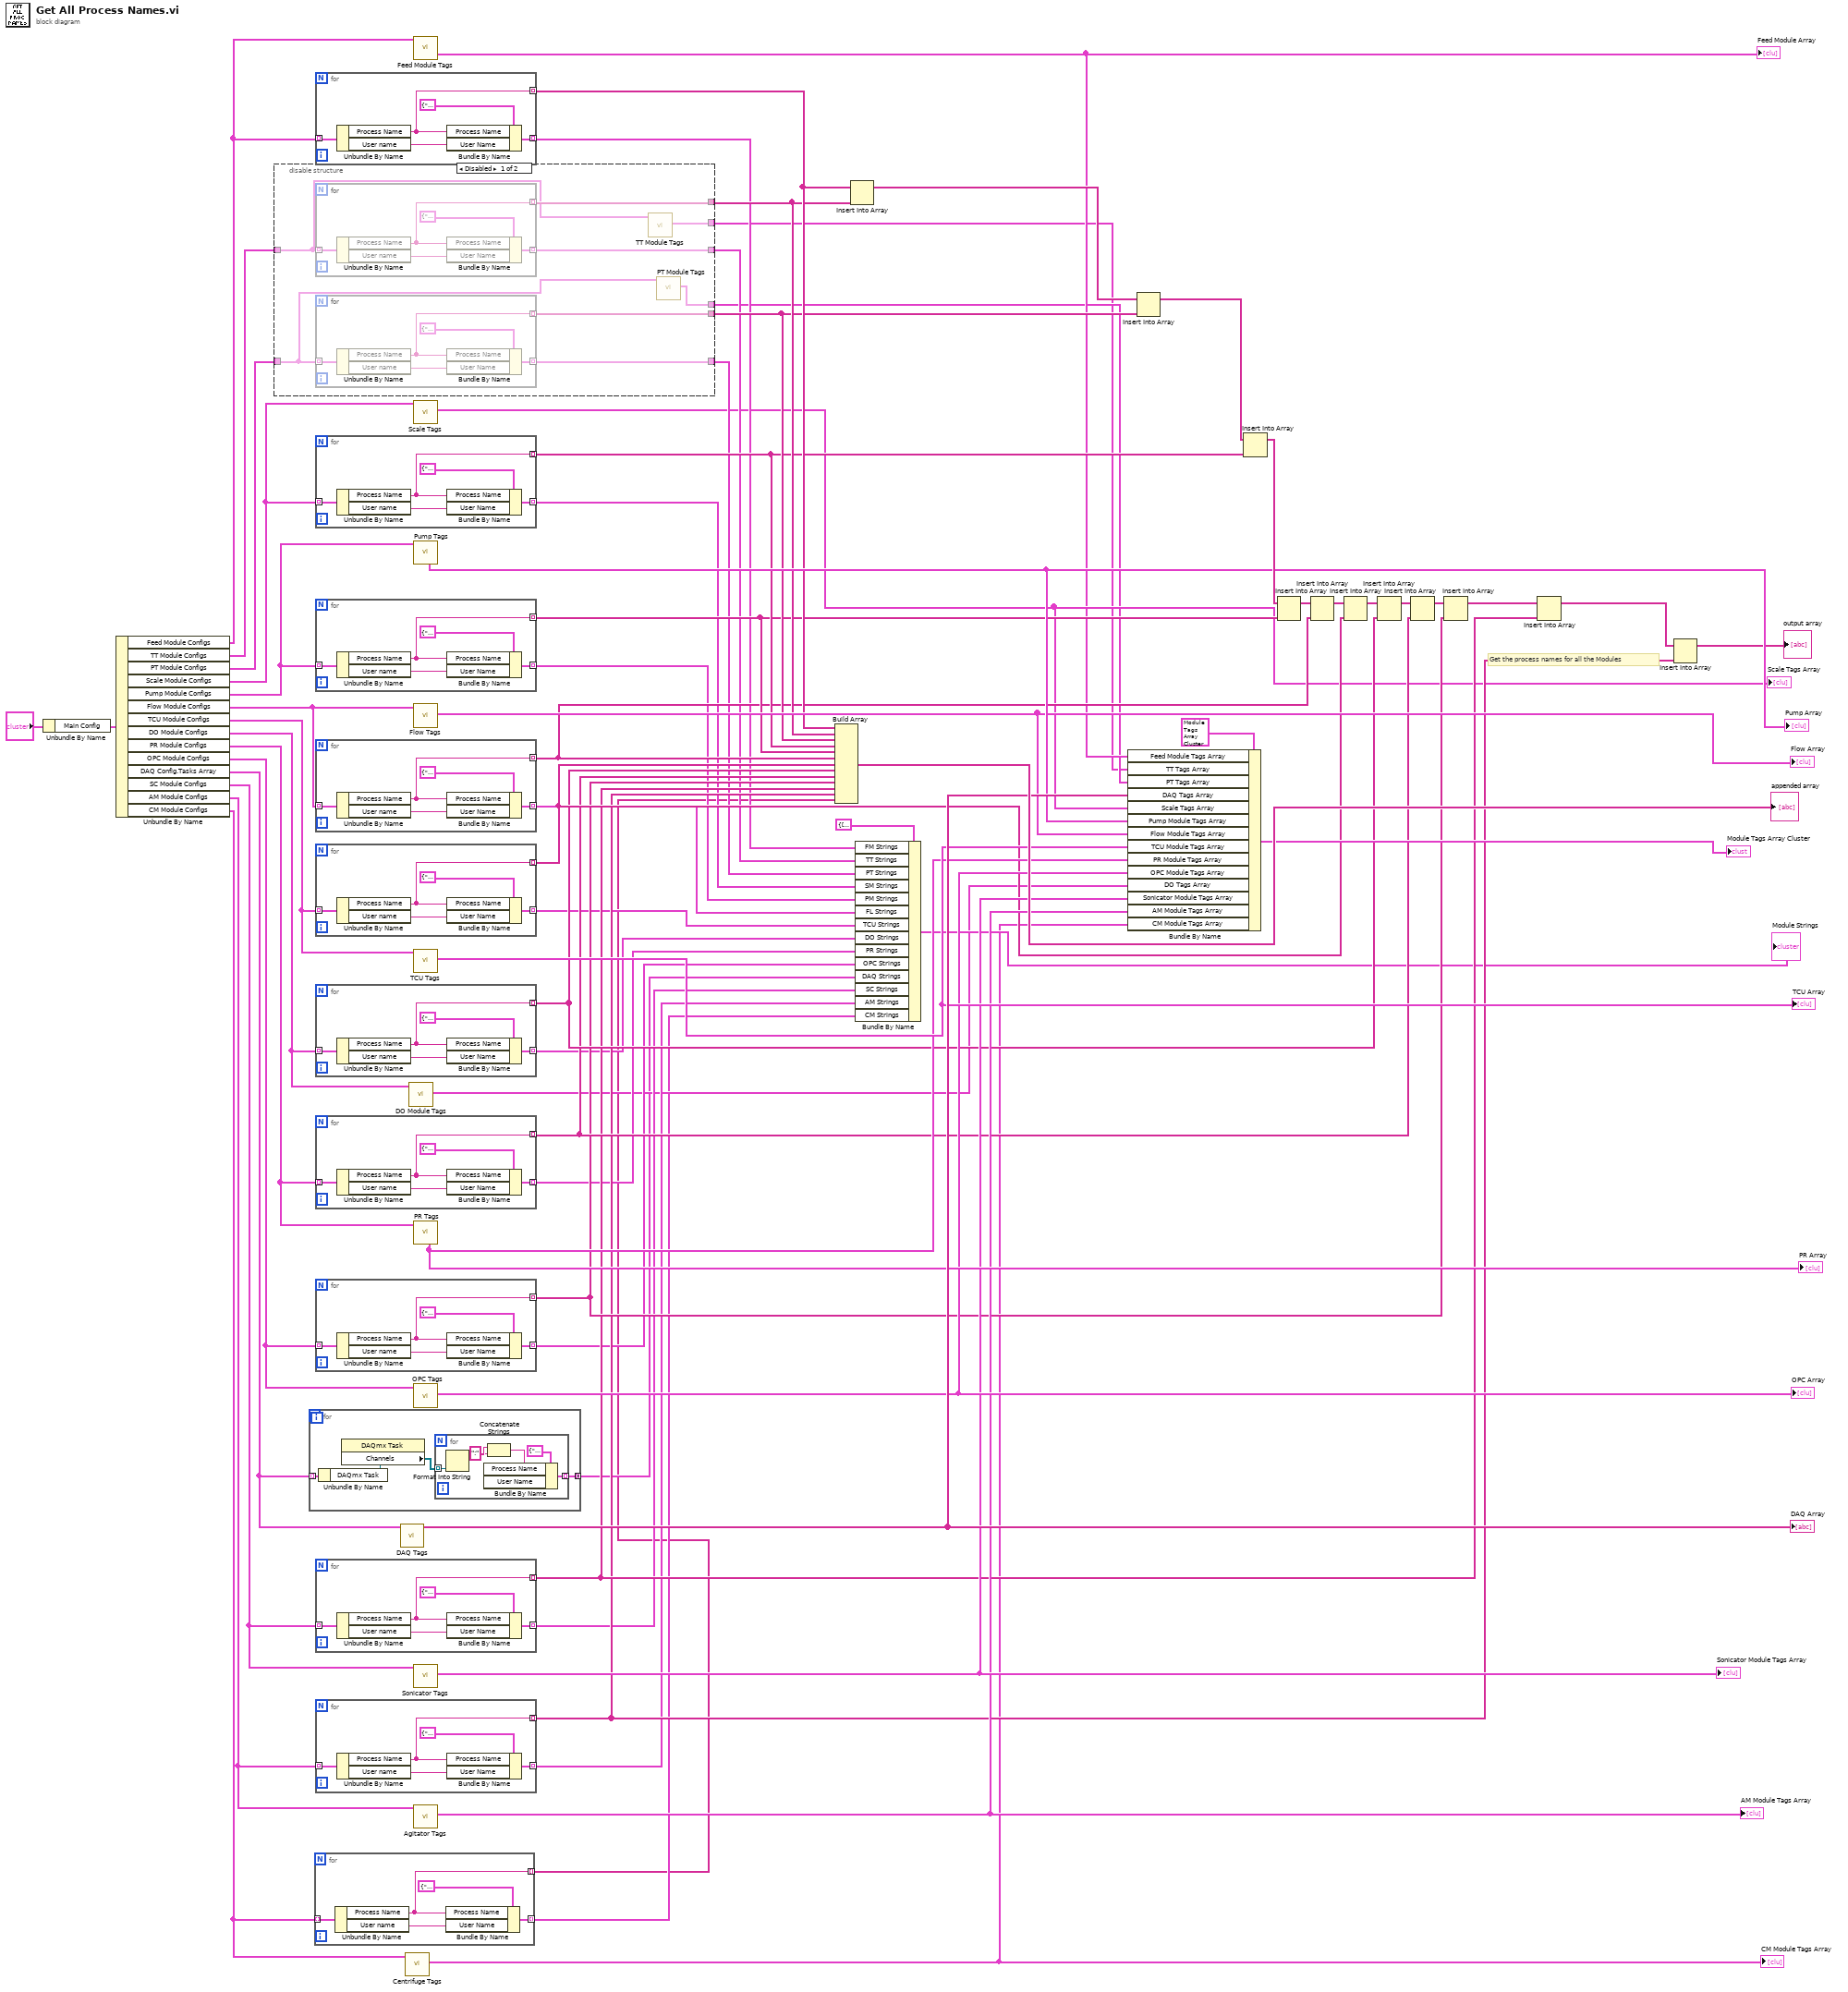
[diagram p0: block diagram]
diagram:
  # "Get the process names for all the Modules"
  n1 = Unbundle By Name("?") -> ("Main Config"=w73:T22)
  n2 = Unbundle By Name(w73) -> ("Feed Module Configs"=w50:T33[], "TT Module Configs"=w16:T53[], "PT Module Configs"=w15:T56[], "Scale Module Configs"=w49:T57[], "Pump Module Configs"=w48:T59[], "Flow Module Configs"=w47:T63[], "TCU Module Configs"=w46:T65[], "DO Module Configs"=w14:T74[], "PR Module Configs"=w45:T79[], "OPC Module Configs"=w44:T23[], "DAQ Config.Tasks Array"=w11:T55[], "SC Module Configs"=w43:T83[], "AM Module Configs"=w5:T86[], "CM Module Configs"=w1:T89[])
  n3 = disable-structure shown="Disabled" {
    disable-tunnel: [w81 _] -> w41
    disable-tunnel: [w80 _] -> w40
    disable-tunnel: [w79 _] -> w29
    disable-tunnel: [w78 _] -> w28
    disable-tunnel: w16 -> [w75 _]
    disable-tunnel: w15 -> [w77 _]
    disable-tunnel: [w76 _] -> w7
    disable-tunnel: [w74 _] -> w6
    frame Disabled {
      n4 = for {
        tunnel: w75 -> [w91] mode=indexing
        tunnel: [w88] -> w79 mode=indexing
        tunnel: [w87] -> w81 mode=indexing
        n5 = Unbundle By Name(w91) -> ("Process Name"=w87:string, "User name"=w89:string)
        n6 = Bundle By Name(cluster=T93 {"Process Name"="", "User Name"=""}, "Process Name"=w87, "User Name"=w89) -> (w88:T93)
      }
      n7 = for {
        tunnel: w77 -> [w86] mode=indexing
        tunnel: [w83] -> w78 mode=indexing
        tunnel: [w82] -> w80 mode=indexing
        n8 = Unbundle By Name(w86) -> ("Process Name"=w82:string, "User name"=w84:string)
        n9 = Bundle By Name(cluster=T93 {"Process Name"="", "User Name"=""}, "Process Name"=w82, "User Name"=w84) -> (w83:T93)
      }
      n10 = call "TT Module Tags.vi"("TT Module Config"=w75) -> ("TT Tags Array"=w74:T8[])  [unwired: 9 in, 1 out]
      n11 = call "PT Module Tags.vi"("PT Module Config"=w77) -> ("PT Tags Array"=w76:T9[])  [unwired: 9 in, 1 out]
    }
    frame Enabled {
    }
  }
  n12 = for {
    tunnel: w11 -> [w93] mode=indexing
    tunnel: [w92] -> w8 mode=concatenating
    n13 = Unbundle By Name(w93) -> ("DAQmx Task"=w95:refnum<k21>)
    n14 = property class="DAQmx Task"(reference=w95) -> ("Channels"=w94:refnum<k21>[])  [unwired: 1 in, 2 out]
    n15 = for {
      tunnel: w94 -> [w101] mode=indexing
      tunnel: [w100] -> w92 mode=indexing
      n16 = Format Into String(w101) -> (resulting string=w98:string)  [unwired: 3 in, 1 out]
      n17 = Concatenate Strings(w98, ":" ("string")) -> (w96:string)
      n18 = Bundle By Name(cluster=T93 {"Process Name"="", "User Name"=""}, "Process Name"=w96, "User Name"=w96) -> (w100:T93)
    }
  }
  n19 = for {
    tunnel: w1 -> [w106] mode=indexing
    tunnel: [w103] -> w4 mode=indexing
    tunnel: [w102] -> w3 mode=indexing
    n20 = Unbundle By Name(w106) -> ("Process Name"=w102:string, "User name"=w104:string)
    n21 = Bundle By Name(cluster=T93 {"Process Name"="", "User Name"=""}, "Process Name"=w102, "User Name"=w104) -> (w103:T93)
  }
  n22 = for {
    tunnel: w50 -> [w111] mode=indexing
    tunnel: [w108] -> w30 mode=indexing
    tunnel: [w107] -> w42 mode=indexing
    n23 = Unbundle By Name(w111) -> ("Process Name"=w107:string, "User name"=w109:string)
    n24 = Bundle By Name(cluster=T93 {"Process Name"="", "User Name"=""}, "Process Name"=w107, "User Name"=w109) -> (w108:T93)
  }
  n25 = for {
    tunnel: w49 -> [w116] mode=indexing
    tunnel: [w113] -> w27 mode=indexing
    tunnel: [w112] -> w39 mode=indexing
    n26 = Unbundle By Name(w116) -> ("Process Name"=w112:string, "User name"=w114:string)
    n27 = Bundle By Name(cluster=T93 {"Process Name"="", "User Name"=""}, "Process Name"=w112, "User Name"=w114) -> (w113:T93)
  }
  n28 = for {
    tunnel: w48 -> [w121] mode=indexing
    tunnel: [w118] -> w26 mode=indexing
    tunnel: [w117] -> w38 mode=indexing
    n29 = Unbundle By Name(w121) -> ("Process Name"=w117:string, "User name"=w119:string)
    n30 = Bundle By Name(cluster=T93 {"Process Name"="", "User Name"=""}, "Process Name"=w117, "User Name"=w119) -> (w118:T93)
  }
  n31 = for {
    tunnel: w47 -> [w126] mode=indexing
    tunnel: [w123] -> w25 mode=indexing
    tunnel: [w122] -> w37 mode=indexing
    n32 = Unbundle By Name(w126) -> ("Process Name"=w122:string, "User name"=w124:string)
    n33 = Bundle By Name(cluster=T93 {"Process Name"="", "User Name"=""}, "Process Name"=w122, "User Name"=w124) -> (w123:T93)
  }
  n34 = for {
    tunnel: w46 -> [w131] mode=indexing
    tunnel: [w128] -> w24 mode=indexing
    tunnel: [w127] -> w36 mode=indexing
    n35 = Unbundle By Name(w131) -> ("Process Name"=w127:string, "User name"=w129:string)
    n36 = Bundle By Name(cluster=T93 {"Process Name"="", "User Name"=""}, "Process Name"=w127, "User Name"=w129) -> (w128:T93)
  }
  n37 = for {
    tunnel: w14 -> [w136] mode=indexing
    tunnel: [w133] -> w23 mode=indexing
    tunnel: [w132] -> w35 mode=indexing
    n38 = Unbundle By Name(w136) -> ("Process Name"=w132:string, "User name"=w134:string)
    n39 = Bundle By Name(cluster=T93 {"Process Name"="", "User Name"=""}, "Process Name"=w132, "User Name"=w134) -> (w133:T93)
  }
  n40 = for {
    tunnel: w45 -> [w141] mode=indexing
    tunnel: [w138] -> w22 mode=indexing
    tunnel: [w137] -> w34 mode=indexing
    n41 = Unbundle By Name(w141) -> ("Process Name"=w137:string, "User name"=w139:string)
    n42 = Bundle By Name(cluster=T93 {"Process Name"="", "User Name"=""}, "Process Name"=w137, "User Name"=w139) -> (w138:T93)
  }
  n43 = for {
    tunnel: w44 -> [w146] mode=indexing
    tunnel: [w143] -> w21 mode=indexing
    tunnel: [w142] -> w33 mode=indexing
    n44 = Unbundle By Name(w146) -> ("Process Name"=w142:string, "User name"=w144:string)
    n45 = Bundle By Name(cluster=T93 {"Process Name"="", "User Name"=""}, "Process Name"=w142, "User Name"=w144) -> (w143:T93)
  }
  n46 = for {
    tunnel: w43 -> [w151] mode=indexing
    tunnel: [w148] -> w20 mode=indexing
    tunnel: [w147] -> w32 mode=indexing
    n47 = Unbundle By Name(w151) -> ("Process Name"=w147:string, "User name"=w149:string)
    n48 = Bundle By Name(cluster=T93 {"Process Name"="", "User Name"=""}, "Process Name"=w147, "User Name"=w149) -> (w148:T93)
  }
  n49 = for {
    tunnel: w5 -> [w156] mode=indexing
    tunnel: [w153] -> w19 mode=indexing
    tunnel: [w152] -> w31 mode=indexing
    n50 = Unbundle By Name(w156) -> ("Process Name"=w152:string, "User name"=w154:string)
    n51 = Bundle By Name(cluster=T93 {"Process Name"="", "User Name"=""}, "Process Name"=w152, "User Name"=w154) -> (w153:T93)
  }
  n52 = call "DAQ Tags.vi"("Tasks"=w11) -> ("DAQ Tags Array"=w62:string[])  [unwired: 10 in]
  "DAQ Array" <- w62
  n53 = call "Centrifuge Tags.vi"("AM Module Configs"=w1) -> ("CM Module Tags Array"=w2:T1[])  [unwired: 7 in, 3 out]
  "CM Module Tags Array" <- w2
  n54 = call "DO Module Tags.vi"("DO Module Config"=w14) -> ("DO Tags Array"=w13:T13[])  [unwired: 9 in, 1 out]
  n55 = call "Feed Module Tags.vi"("Feed Module Configs"=w50) -> ("Feed Module Tags Array"=w12:T7[])  [unwired: 6 in, 8 out]
  "Feed Module Array" <- w12
  n56 = call "Scale Tags.vi"("Scale Module Configs"=w49) -> ("Scale Tags Array"=w17:T2)  [unwired: 8 in, 2 out]
  "Scale Tags Array" <- w17
  n57 = call "Pump Tags.vi"("Pump Module Configs"=w48) -> ("Pump Module Tags Array"=w61:T10[])  [unwired: 7 in, 3 out]
  "Pump Array" <- w61
  n58 = call "Flow Tags.vi"("Flow Module Configs"=w47) -> ("Flow Module Tags Array"=w60:T11[])  [unwired: 7 in, 3 out]
  "Flow Array" <- w60
  n59 = call "TCU Tags.vi"("TCU Module Configs"=w46) -> ("TCU Module Tags Array"=w59:T12[])  [unwired: 7 in, 3 out]
  "TCU Array" <- w59
  n60 = call "PR Tags.vi"("PR Module Configs"=w45) -> ("PR Module Tags Array"=w58:T14[])  [unwired: 6 in, 4 out]
  "PR Array" <- w58
  n61 = call "OPC Tags.vi"("OPC Module Configs"=w44) -> ("OPC Module Tags Array"=w57:T15[])  [unwired: 7 in, 3 out]
  "OPC Array" <- w57
  n62 = call "Sonicator Tags.vi"("SC Module Configs"=w43) -> ("Sonicator Module Tags Array"=w52:T5[])  [unwired: 8 in, 2 out]
  "Sonicator Module Tags Array" <- w52
  n63 = call "Agitator Tags.vi"("AM Module Configs"=w5) -> ("AM Module Tags Array"=w51:T4[])  [unwired: 7 in, 3 out]
  "AM Module Tags Array" <- w51
  n64 = Build Array(w42, w41, w40, w39, w38, w37, w36, w35, w34, w33, w32, w31, w3) -> (→"appended array":string[][])
  n65 = Insert Into Array(array=w42, new element=w41) -> (w70:string[])  [unwired: 1 in]
  n66 = Bundle By Name(cluster=T3 {"FM Strings"=[], "TT Strings"=[], "PT Strings"=[], "SM Strings"=[], "PM Strings"=[], "FL Strings"=[], "TCU Strings"=[], "DO Strings"=[], "PR Strings"=[], "OPC Strings"=[], "DAQ Strings"=[], "SC Strings"=[], "AM Strings"=[], "CM Strings"=[]} ("Module Strings 2"), "FM Strings"=w30, "TT Strings"=w29, "PT Strings"=w28, "SM Strings"=w27, "PM Strings"=w26, "FL Strings"=w25, "TCU Strings"=w24, "DO Strings"=w23, "PR Strings"=w22, "OPC Strings"=w21, "DAQ Strings"=w8, "SC Strings"=w20, "AM Strings"=w19, "CM Strings"=w4) -> (→"Module Strings":T3)
  n67 = Bundle By Name(cluster=T6 {"Feed Module Tags Array"=[], "TT Tags Array"=[], "PT Tags Array"=[], "DAQ Tags Array"=[], "Scale Tags Array"=[], "Pump Module Tags Array"=[], "Flow Module Tags Array"=[], "TCU Module Tags Array"=[], "DO Tags Array"=[], "PR Module Tags Array"=[], "OPC Module Tags Array"=[], "Sonicator Module Tags Array"=[], "AM Module Tags Array"=[], "CM Module Tags Array"=[]} ("Module Tags Array Cluster"), "Feed Module Tags Array"=w12, "TT Tags Array"=w6, "PT Tags Array"=w7, "DAQ Tags Array"=w62, "Scale Tags Array"=w17, "Pump Module Tags Array"=w61, "Flow Module Tags Array"=w60, "TCU Module Tags Array"=w59, "PR Module Tags Array"=w58, "OPC Module Tags Array"=w57, "DO Tags Array"=w13, "Sonicator Module Tags Array"=w52, "AM Module Tags Array"=w51, "CM Module Tags Array"=w2) -> (→"Module Tags Array Cluster":T6)
  n68 = Insert Into Array(array=w70, new element=w40) -> (w69:string[])  [unwired: 1 in]
  n69 = Insert Into Array(array=w69, new element=w39) -> (w68:string[])  [unwired: 1 in]
  n70 = Insert Into Array(array=w68, new element=w38) -> (w67:string[])  [unwired: 1 in]
  n71 = Insert Into Array(array=w67, new element=w37) -> (w66:string[])  [unwired: 1 in]
  n72 = Insert Into Array(array=w66, new element=w36) -> (w65:string[])  [unwired: 1 in]
  n73 = Insert Into Array(array=w65, new element=w35) -> (w64:string[])  [unwired: 1 in]
  n74 = Insert Into Array(array=w64, new element=w34) -> (w63:string[])  [unwired: 1 in]
  n75 = Insert Into Array(array=w63, new element=w33) -> (w55:string[])  [unwired: 1 in]
  n76 = Insert Into Array(array=w55, new element=w32) -> (w54:string[])  [unwired: 1 in]
  n77 = Insert Into Array(array=w54, new element=w31) -> (→"output array":string[])  [unwired: 1 in]
